vi "Main.vi"() -> ()   [LabVIEW 2016]
doc: "The myRIO Project template acquires acceleration data from the onboard accelerometer and displays the changes of acceleration values in a waveform chart."
uses:
  <vilib>/FPGAPlugInAG/myRIO-1900/niLvFpga_Open_myRIO-1900.vi
  <vilib>/rvi/interface/common/dynamic/niFpgaDynamicAddResources.vi
  <vilib>/Utility/error.llb/Error Cluster From Error Code.vi
  <vilib>/rvi/errors/niLvFpgaAdjustHostInterfaceError.vi
  <vilib>/FPGAPlugInAG/Dynamic/niLvFpga_Close_Dynamic.vi
  <vilib>/rvi/interface/nirviOpenFPGA/nirviOpenFPGA.xnode
  FPGA Bitfiles/WS2811driver_FPGATarget_FPGAmain_HaK4FqHt+Z8.lvbitx
  <vilib>/rvi/interface/nirviReadWriteControl/nirviReadWriteControl.xnode
  <vilib>/rvi/interface/nirviCloseFPGA/nirviCloseFPGA.xnode
  NiFpgaLv.dll
  <vilib>/rvi/interface/Simulation/niFpgaSimulationCallBeginRW.vi
panel:
  in  "reset ticks)":u32=2000
  in  "number of leds":i32=1
  in  "Array":bool[](array[boolean])=[FALSE, FALSE, FALSE, FALSE, FALSE, FALSE, FALSE, TRUE, FALSE, FALSE, FALSE, FALSE, FALSE, FALSE, FALSE, FALSE, FALSE, FALSE, FALSE, FALSE, FALSE, FALSE, FALSE, FALSE]
  in  "Stop Button":bool
  out "error out":errorcluster
  # "Overview: The myRIO Project template acquires acceleration data from the onboard accelerometer and displays the changes of acceleration values in a waveform chart.\nInstructions:\n1. Check the myRIO target IP address in the project and make sure the target IP address is correct. \n2. Run this VI."
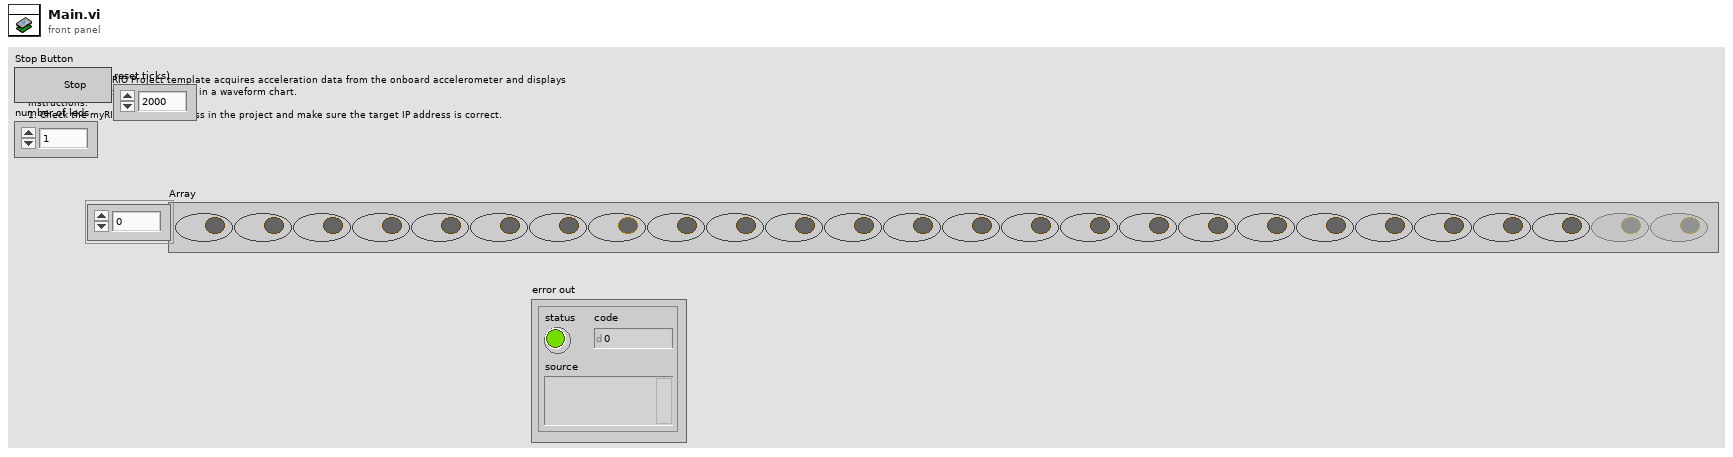
[diagram p1: front panel]
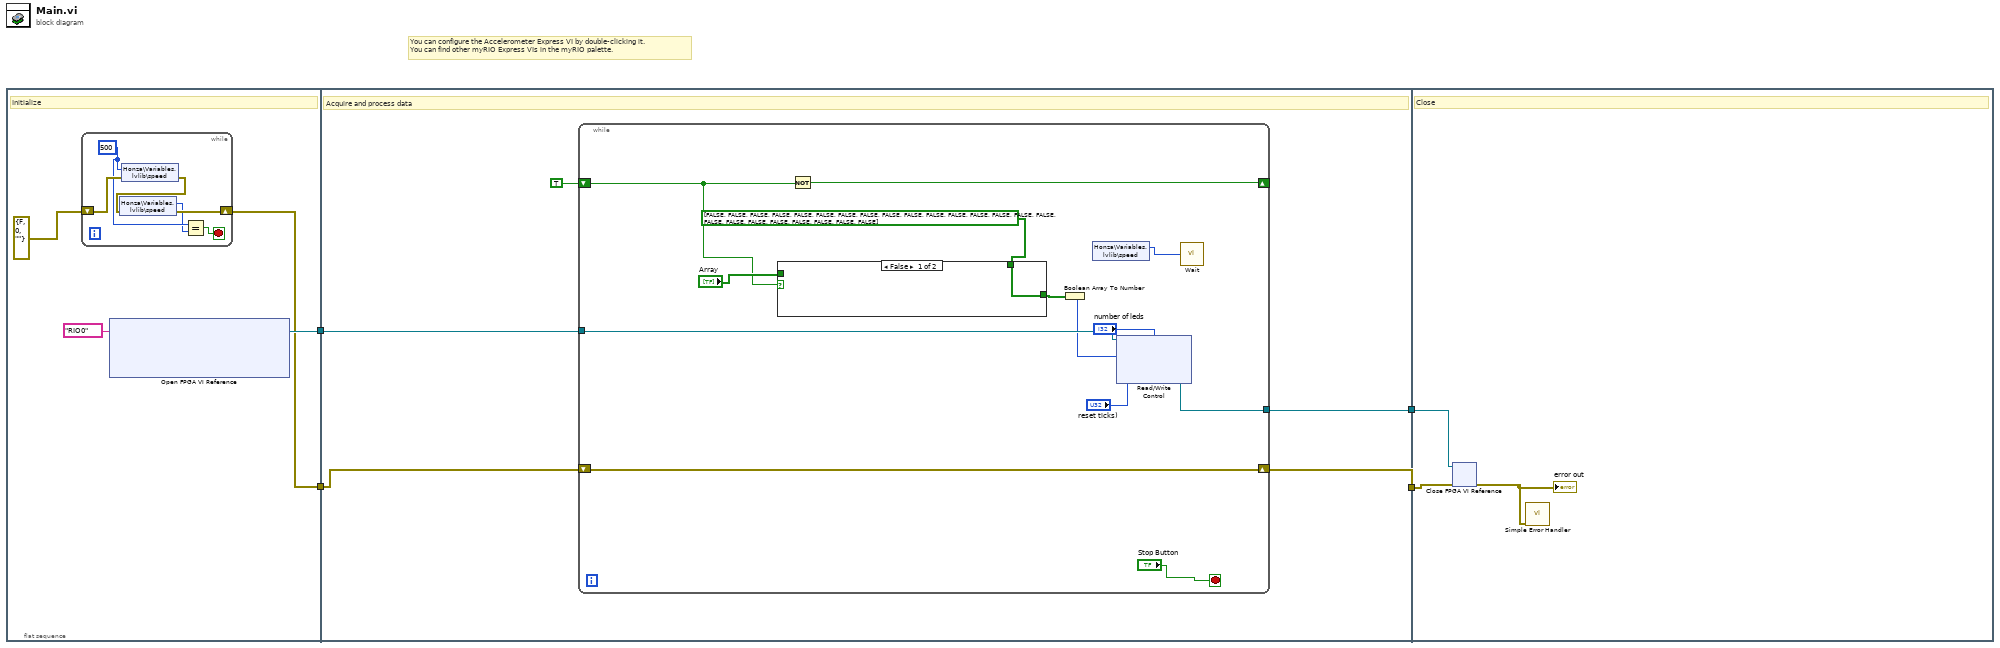
[diagram p0: block diagram]
diagram:
  # "You can configure the Accelerometer Express VI by double-clicking it.\nYou can find other myRIO Express VIs in the myRIO palette."
  n1 = flat-sequence {
    tunnel: [w6] -> w4
    tunnel: [w8] -> w2
    tunnel: w4 -> [w18]
    tunnel: [w19] -> w3
    tunnel: w2 -> [w17]
    tunnel: [w16] -> w1
    tunnel: w3 -> [w37]
    tunnel: w1 -> [w35]
    frame #0 {
      # "Initialize"
      n2 = while {
        shift-right: [w14] -> w6
        shift-left: errorcluster {"status"=FALSE, "code"=0, "source"=""} ("error in (no error)") -> [w13]
        stop <- w11 stop-if-true
        w10 = 500 ("speed")
        n3 = shared-variable "Honza\\Variables.lvlib\\speed"(w10, error in=w13) -> (error out=w12:errorcluster)
        n4 = shared-variable "Honza\\Variables.lvlib\\speed"(error in=w12) -> (w9:i32, error out=w14:errorcluster)
        n5 = Equal?(x=w10, y=w9) -> (x = y?=w11:bool)
      }
      n6 = xnode "Open FPGA VI Reference"("resource name"=tag "RIO0") -> ("FPGA VI Reference Out"=w8:refnum<k20>)  [unwired: 1 in, 1 out]
    }
    frame #1 {
      # "Acquire and process data"
      n7 = while {
        shift-right: [w27] -> w19
        shift-left: w18 -> [w27]
        tunnel: w17 -> [w32]
        tunnel: [w30] -> w16
        shift-right: [w23] -> _
        shift-left: TRUE -> [w20]
        stop <- "Stop Button" stop-if-true
        n8 = case shown="False" w20 {
          tunnel: [w33 w34] -> w28
          tunnel: bool[] [FALSE, FALSE, FALSE, FALSE, FALSE, FALSE, FALSE, FALSE, FALSE, FALSE, FALSE, FALSE, FALSE, FALSE, FALSE, FALSE, FALSE, FALSE, FALSE, FALSE, FALSE, FALSE, FALSE, FALSE] ("Array") -> [w33 _]
          tunnel: "Array" -> [_ w34]
          frame False {
          }
          frame True {
          }
        }
        n9 = Not(x=w20) -> (.not. x?=w23:bool)
        n10 = Boolean Array To Number(Boolean array=w28) -> (number=w29:u32)
        n11 = shared-variable "Honza\\Variables.lvlib\\speed"() -> (w24:i32)  [unwired: 1 in, 1 out]
        n12 = xnode "Read/Write Control"("FPGA VI Reference In"=w32, "color"=w29, "number of leds"="number of leds", "reset ticks)"="reset ticks)") -> ("FPGA VI Reference Out"=w30:refnum<k20>)  [unwired: 1 in, 1 out]
        n13 = call "Wait"("Count(mSec)"=w24) -> ()  [unwired: 1 out]
      }
    }
    frame #2 {
      # "Close"
      n14 = xnode "Close FPGA VI Reference"("FPGA VI Reference In"=w35, "error in"=w37) -> ("error out"=w36:errorcluster)
      "error out" <- w36
      n15 = call <vilib>:"Simple Error Handler.vi"("error in (no error)"=w36) -> ()  [unwired: 4 in, 5 out]
    }
  }
